vi "Sr530 VisaRW.vi"(0 "VISA Rsrc":refnum<visa-resource-name>="SR530", 1 "2Lecture?":bool, 2 "EOS (Aucun)":string, 3 "Délais (0 ms)":u32, 5 "ChaineCom":string caption="Chaîne de commande", 9 "Nbcaract":u32=100 caption="Nombre de \ncaractères à lire", 11 "error in (no error)":errorcluster, 12 "Lecture?(T)":bool=TRUE) -> (4 "VISA Rsrc Out":refnum<visa-resource-name>="GPIB0::12::INSTR", 6 "ChaineRep":string caption="Chaîne de réponse", 8 "ChaineRep2":string caption="Chaîne de réponse 2", 10 "Count out 2":u32=44 caption="Nombre de caractères lus 2", 14 "Count out":u32=44 caption="Nombre de caractères lus", 15 "error out":errorcluster)   [LabVIEW 2019]
doc: "Ce VI envoie des commande d'écriture et de lecture VISA à l'appareil GPIB. Il permet de ne pas séparer un question de sa réponse. Pour que cela fonctionne toute lecture d'un instrument doit se faire par ce VI."
panel:
  out "readTime":u32
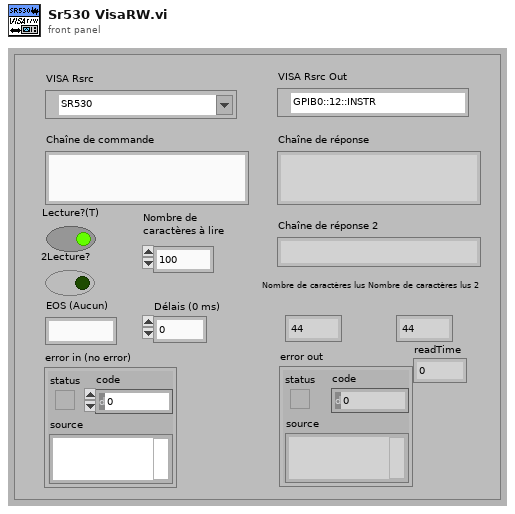
[diagram p1: front panel]
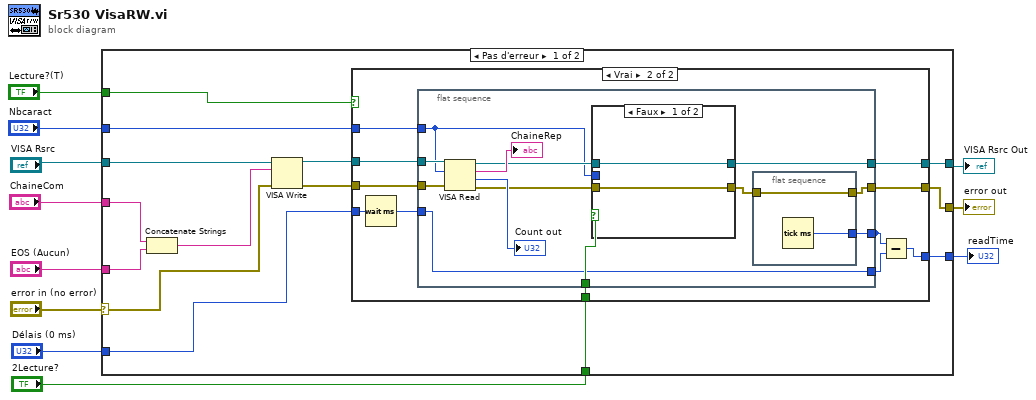
[diagram p0: block diagram]
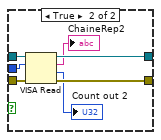
[diagram p3: hidden frame]
diagram:
  n1 = case shown="Pas d'erreur" "error in (no error)" {
    selector: "error in (no error)" -> [w19 w64]
    tunnel: "VISA Rsrc" -> [w20 w63]
    tunnel: [w25 w63] -> w3
    tunnel: "ChaineCom" -> [w24 _]
    tunnel: "EOS (Aucun)" -> [w23 _]
    tunnel: "Délais (0 ms)" -> [w16 _]
    tunnel: "Nbcaract" -> [w15 _]
    tunnel: "Lecture?(T)" -> [w14 _]
    tunnel: [w21 w64] -> w5
    tunnel: "2Lecture?" -> [w13 _]
    tunnel: [w12 _] -> w1
    frame No Error {
      n2 = Concatenate Strings(w24, w23) -> (w22:string)
      n3 = VISA Write(VISA resource name=w20, write buffer=w22, error in (no error)=w19) -> (VISA resource name out=w18:refnum<visa-resource-name>, error out=w17:errorcluster)  [unwired: 1 out]
      n4 = case shown="Vrai" w14 {
        tunnel: w18 -> [w27 w38]
        tunnel: [w27 w37] -> w25
        tunnel: w17 -> [w26 w36]
        tunnel: [w26 w35] -> w21
        tunnel: w15 -> [_ w34]
        tunnel: w16 -> [_ w33]
        tunnel: w13 -> [_ w31]
        tunnel: [_ w28] -> w12
        frame False {
        }
        frame True {
          n5 = Wait (ms)(milliseconds to wait=w33) -> (millisecond timer value=w32:u32)
          n6 = flat-sequence {
            tunnel: [w42] -> w35
            tunnel: [w45] -> w37
            tunnel: w38 -> [w51]
            tunnel: w36 -> [w49]
            tunnel: w34 -> [w43]
            tunnel: w32 -> [w40]
            tunnel: w31 -> [w44]
            tunnel: [w40] -> w29
            tunnel: [w39] -> _
            tunnel: [w39] -> w30
            frame #0 {
              n7 = VISA Read(VISA resource name=w51, byte count=w43, error in (no error)=w49) -> (VISA resource name out=w46:refnum<visa-resource-name>, read buffer=→"ChaineRep":string, return count=→"Count out":u32, error out=w47:errorcluster)
              n8 = case shown="Faux" w44 {
                tunnel: w47 -> [w54 w62]
                tunnel: [w54 w61] -> w41
                tunnel: w46 -> [w55 w60]
                tunnel: [w55 w59] -> w45
                tunnel: w43 -> [_ w56]
                frame False {
                }
                frame True {
                  n9 = VISA Read(VISA resource name=w60, byte count=w56, error in (no error)=w62) -> (VISA resource name out=w59:refnum<visa-resource-name>, read buffer=→"ChaineRep2":string, return count=→"Count out 2":u32, error out=w61:errorcluster)
                }
              }
              n10 = flat-sequence {
                tunnel: [w53] -> w42
                tunnel: w41 -> [w53]
                tunnel: [w52] -> w39
                frame #0 {
                  n11 = Tick Count (ms)() -> (millisecond timer value=w52:u32)
                }
              }
            }
          }
          n12 = Subtract(x=w30, y=w29) -> (x-y=w28:u32)
        }
      }
    }
    frame Error {
    }
  }
  "error out" <- w5
  "VISA Rsrc Out" <- w3
  "readTime" <- w1
